vi "Files Classification_V5.vi"() -> ()   [LabVIEW 2022 SP3]
uses:
  <vilib>/Utility/file.llb/Read Delimited Spreadsheet (DBL).vi
  <vilib>/Utility/file.llb/Write Delimited Spreadsheet (DBL).vi
panel:
  in  "Sampling Range (nm):":string(combo)="5"
  out "完成進度(%)":dbl(slide) scale=0.0..100.0
  out "New path":path
  out "Hours  2":dbl
  out "Minutes":dbl
  out "Seconds  2":dbl
  in  "Choose an arbitrary file":path
  in  "End (nm) :":dbl=700.0
  in  "Start (nm) :":dbl=400.0
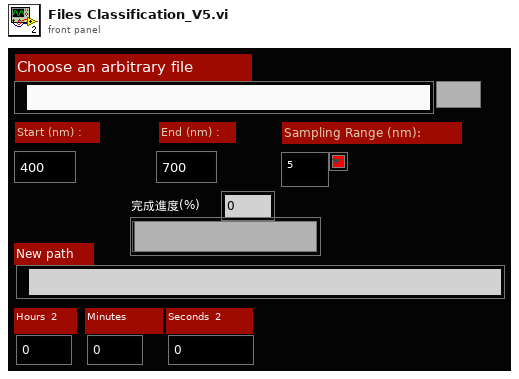
[diagram p1: front panel]
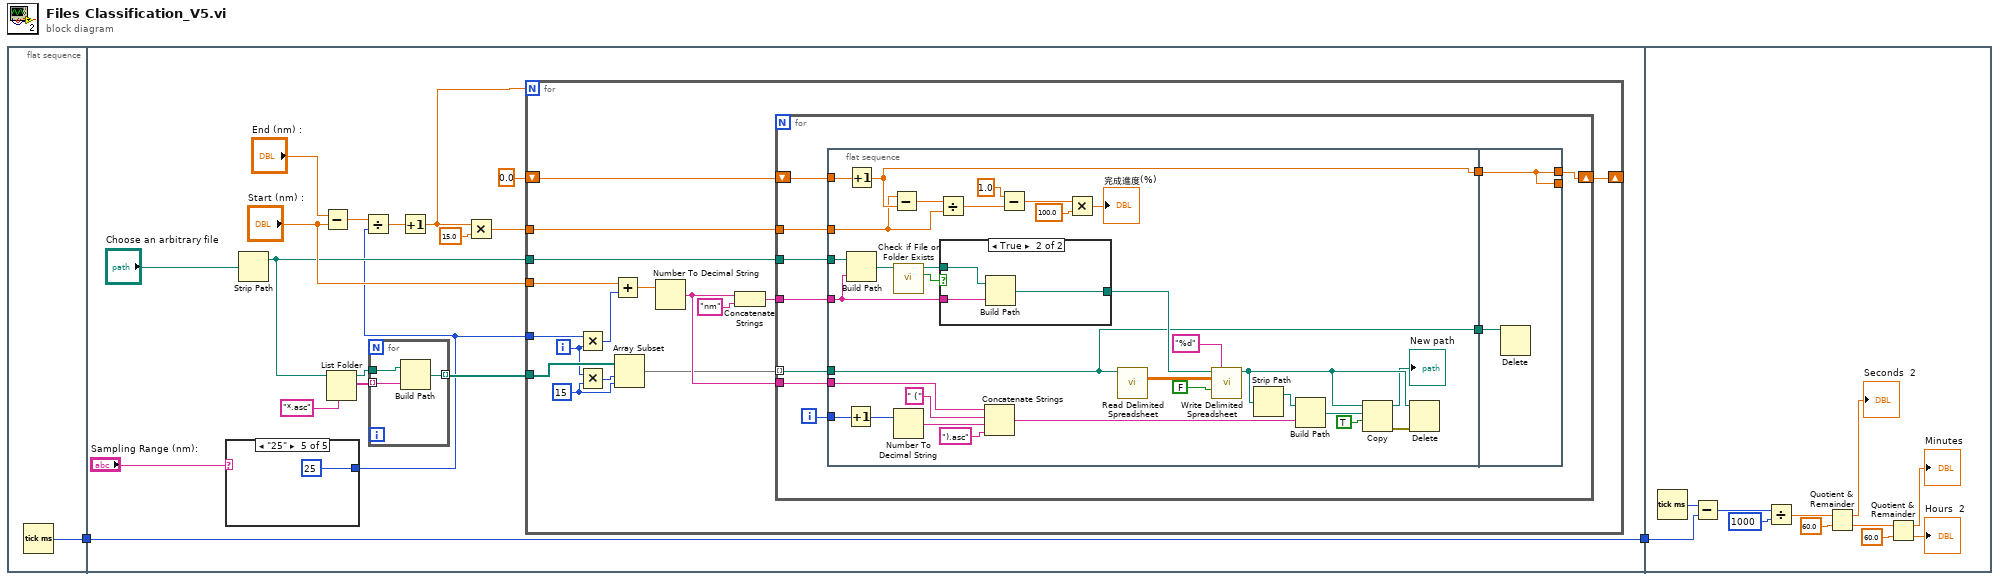
[diagram p0: block diagram]
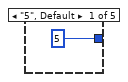
[diagram p2: hidden frame]
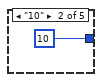
[diagram p3: hidden frame]
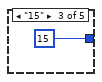
[diagram p4: hidden frame]
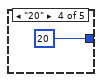
[diagram p5: hidden frame]
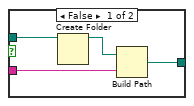
[diagram p6: hidden frame]
diagram:
  n1 = flat-sequence {
    tunnel: [w3] -> w1
    tunnel: [w10] -> w2
    tunnel: w1 -> [w10]
    tunnel: w2 -> [w96]
    frame #0 {
      n2 = Tick Count (ms)() -> (millisecond timer value=w3:u32)
    }
    frame #1 {
      n3 = case shown="\"25\"" "Sampling Range (nm):" {
        tunnel: [i8 5 i8 10 i8 15 i8 20 i8 25] -> w4
        frame "5", Default {
        }
        frame "10" {
        }
        frame "15" {
        }
        frame "20" {
        }
        frame "25" {
        }
      }
      n4 = Strip Path(path="Choose an arbitrary file") -> (stripped path=w11:path)  [unwired: 1 out]
      n5 = Subtract(x="End (nm) :", y="Start (nm) :") -> (x-y=w19:dbl)
      n6 = List Folder(path=w11, pattern="*.asc") -> (path out=w15:path, filenames=w16:string[])  [unwired: 2 in, 2 out]
      n7 = Divide(x=w19, y=w4) -> (x/y=w20:dbl)
      n8 = for {
        tunnel: w16 -> [w94] mode=indexing
        tunnel: w15 -> [w95]
        tunnel: [w93] -> w12 mode=indexing
        n9 = Build Path(base path=w95, name or relative path=w94) -> (appended path=w93:path)
      }
      n10 = Increment(x=w20) -> (x+1=w8:dbl)
      n11 = Multiply(x=w8, y=15.0) -> (x*y=w7:dbl)
      n12 = for {
        N: w8 -> [_]
        tunnel: w4 -> [w41]
        tunnel: "Start (nm) :" -> [w39]
        tunnel: w11 -> [w34]
        tunnel: w12 -> [w33]
        tunnel: w7 -> [w28]
        shift-right: [w26] -> _
        shift-left: 0.0 -> [w27]
        i -> [w32]
        w31 = 15 ("length")
        n13 = Multiply(x=w41, y=w32) -> (x*y=w40:i32)
        n14 = Multiply(x=w32, y=w31) -> (x*y=w30:i32)
        n15 = Add(x=w39, y=w40) -> (x+y=w38:dbl)
        n16 = Array Subset(array=w33, index=w30, length=w31) -> (w29:path[])
        n17 = Number To Decimal String(number=w38) -> (decimal integer string=w36:string)  [unwired: 1 in]
        n18 = Concatenate Strings(w36, "nm") -> (w35:string)
        n19 = for {
          tunnel: w36 -> [w51]
          tunnel: w35 -> [w47]
          tunnel: w34 -> [w49]
          tunnel: w29 -> [w48] mode=indexing
          shift-right: [w43] -> w26
          shift-left: w27 -> [w45]
          tunnel: w28 -> [w42]
          i -> [w50]
          n20 = flat-sequence {
            tunnel: w51 -> [w83]
            tunnel: w50 -> [w82]
            tunnel: w49 -> [w71]
            tunnel: w48 -> [w63]
            tunnel: w47 -> [w64]
            tunnel: [w63] -> w46
            tunnel: w45 -> [w60]
            tunnel: [w59] -> w44
            tunnel: w42 -> [w57]
            tunnel: w46 -> [w92]
            tunnel: w44 -> [w91]
            tunnel: [w91] -> _
            tunnel: [w91] -> w43
            frame #0 {
              n21 = Increment(x=w82) -> (x+1=w81:i32)
              n22 = Increment(x=w60) -> (x+1=w59:dbl)
              n23 = Build Path(base path=w71, name or relative path=w64) -> (appended path=w72:path)
              n24 = Subtract(x=w57, y=w59) -> (x-y=w58:dbl)
              n25 = call <vilib>:"Check if File or Folder Exists.vi"("path"=w72) -> ("file or folder exists?"=w73:bool, "dup path"=w74:path)  [unwired: 8 in, 1 out]
              n26 = Number To Decimal String(number=w81) -> (decimal integer string=w80:string)  [unwired: 1 in]
              n27 = Divide(x=w58, y=w57) -> (x/y=w54:dbl)
              n28 = case shown="True" w73 {
                tunnel: w74 -> [w87 w90]
                tunnel: [w86 w89] -> w68
                tunnel: w64 -> [w84 w88]
                frame False {
                  n29 = Create Folder(path (use dialog)=w87) -> (created path=w85:path)  [unwired: 2 in, 2 out]
                  n30 = Build Path(base path=w85, name or relative path=w84) -> (appended path=w86:path)
                }
                frame True {
                  n31 = Build Path(base path=w90, name or relative path=w88) -> (appended path=w89:path)
                }
              }
              n32 = Concatenate Strings(w83, " (" ("string"), w80, ").asc" ("string")) -> (w69:string)
              n33 = Subtract(x=1.0, y=w54) -> (x-y=w52:dbl)
              n34 = Multiply(x=w52, y=100.0) -> (x*y=→"完成進度(%)":dbl)
              n35 = call-poly <vilib>:"Read Delimited Spreadsheet.vi"("file path (dialog if empty)"=w63) -> ("all rows"=w66:dbl[][])  [unwired: 9 in, 5 out]
              n36 = call-poly <vilib>:"Write Delimited Spreadsheet.vi"("file path (dialog if empty)"=w68, "format (%.3f)"="%d", "2D data"=w66, "append to file? (new file:F)"=FALSE) -> ("new file path (Not A Path if cancelled)"=w67:path)  [unwired: 10 in, 1 out]
              n37 = Strip Path(path=w67) -> (stripped path=w76:path)  [unwired: 1 out]
              n38 = Build Path(base path=w76, name or relative path=w69) -> (appended path=w75:path)
              n39 = Copy(9:TRUE ("overwrite (F)"), 10:w75, 11:w67) -> (0:w77:errorcluster, 3:→"New path":path)  [unwired: 2 in, 1 out]
              n40 = Delete(path (use dialog)=w67, error in=w77) -> ()  [unwired: 3 in, 3 out]
            }
            frame #1 {
              n41 = Delete(path (use dialog)=w92) -> ()  [unwired: 4 in, 3 out]
            }
          }
        }
      }
    }
    frame #2 {
      n42 = Tick Count (ms)() -> (millisecond timer value=w103:u32)
      n43 = Subtract(x=w103, y=w96) -> (x-y=w104:u32)
      n44 = Divide(x=w104, y=u32 1000) -> (x/y=w105:dbl)
      n45 = Quotient & Remainder(x=w105, y=60.0) -> (x-y*floor(x/y)=→"Seconds  2":dbl, floor(x/y)=w106:dbl)
      n46 = Quotient & Remainder(x=w106, y=60.0) -> (x-y*floor(x/y)=→"Minutes":dbl, floor(x/y)=→"Hours  2":dbl)
    }
  }
